vi "Set Dialog Behavior.vi"(8 "error in":errorcluster, 11 "Flex Dialog in":refnum<class "Flex UI Dialog.lvclass">) -> (0 "error out":errorcluster, 3 "Flex Dialog out":refnum<class "Flex UI Dialog.lvclass">)   [LabVIEW 2016, in "Flex UI Dialog.lvclass"]
doc: "Set the Dialog Behavior."
uses:
  Flex UI Dialog.lvclass
  C:/VI Packages/Flex UI/Flex UI (Parent)/Flex UI.lvclass
  Flex UI (Parent)/Flex UI.lvclass/Flex UI.ctl
  Flex UI Dialog.lvclass/Flex UI Dialog.ctl
  Flex UI (Parent)/Flex UI.lvclass
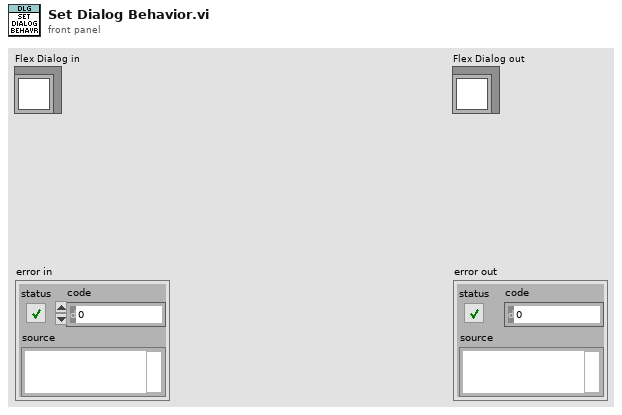
[diagram p1: front panel]
types:
  T1 = enum32{"Invalid", "Default", "Floating", "Floating/Auto-Hide", "Modal"}
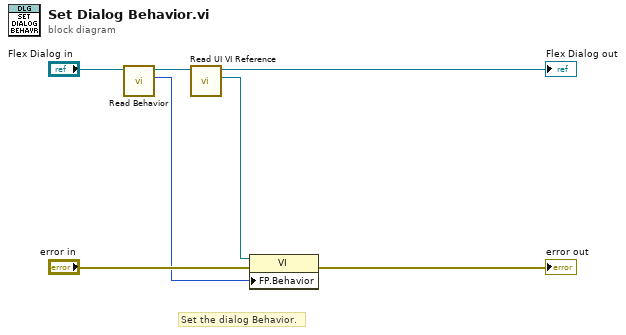
[diagram p0: block diagram]
diagram:
  # "Set the dialog Behavior."
  n1 = call "Read Behavior.vi"("Flex Dialog in"="Flex Dialog in") -> ("Behavior"=w5:T1, "Flex Dialog out"=w2:refnum<class "Flex UI Dialog.lvclass">)  [unwired: 9 in]
  n2 = call "Read UI VI Reference.vi"("Flex UI in"=w2) -> ("UI VI Reference"=w4:refnum<vi>, "Flex UI out"=→"Flex Dialog out":refnum<class "Flex UI Dialog.lvclass">)  [unwired: 9 in]
  n3 = property class="VI"(reference=w4, error in="error in", "FP.Behavior"=w5) -> (error out=→"error out":errorcluster)  [unwired: 1 out]
